vi "Generate Pulse Indexies.vi"(4 "dt":dbl, 5 "Size":i32, 6 "t0":timestamp, 7 "Delay":dbl format="%#_6p", 11 "I-V parameters":T1={"Start magnitude"=0.01, "Magnitude increment"=0.001, "Number of pulses"=8, "Baseline length"=480, "Ramp length"=32, "Top  length"=480, "Threshold "=1e-05, "Processing Delay"=255, "Valhalla range"=0.001, "Interpolation"=64} {"Valhalla range" format="%#_6pA"; "Processing Delay" format="%dpts"; "Threshold" format="%#_6pV"; "Top  length" format="%dpts"; "Ramp length" format="%dpts"; "Baseline length" format="%dpts"; "Magnitude increment" format="%#_6pA"; "Start magnitude" format="%#_6pA"}) -> (3 "Pulse indexies out":T2[](array[typedef]))   [LabVIEW 2016]
uses:
  Pulse indexies.ctl
  I-V parameters.ctl
panel:
  out "32bit integer 2":i32
  out "result":i32
  out "32bit integer":T3
  in  "Pulse indexies":T2
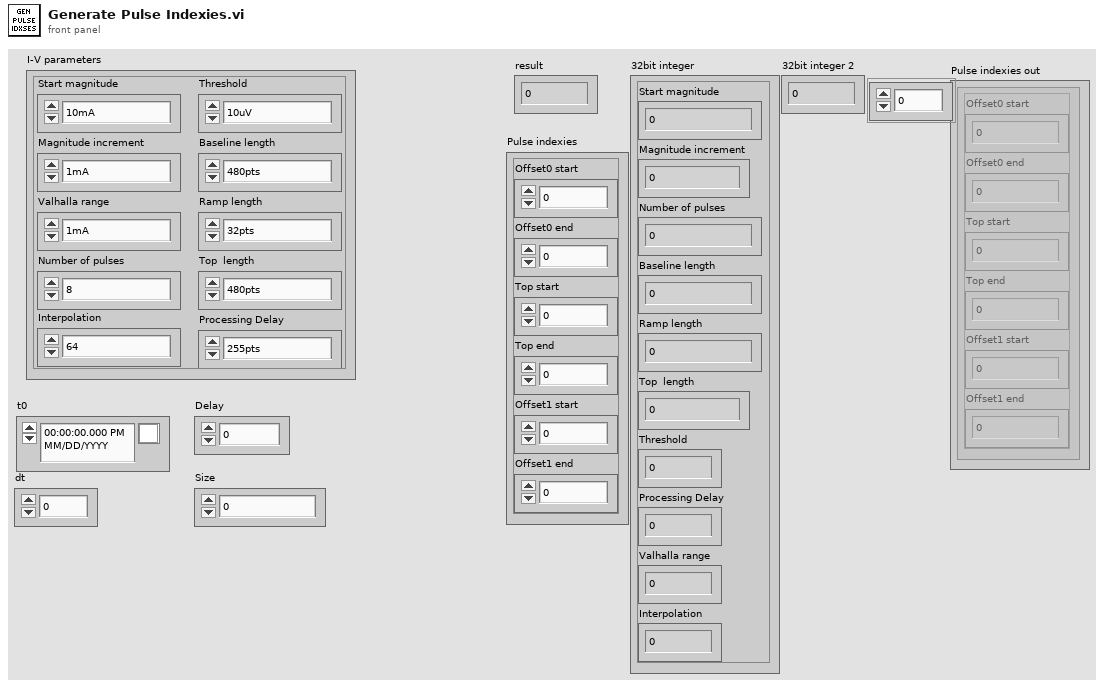
[diagram p1: front panel]
types:
  T1 = typedef "I-V parameters.ctl" = cluster{"Start magnitude":dbl, "Magnitude increment":dbl, "Number of pulses":i32, "Baseline length":i32, "Ramp length":i32, "Top  length":i32, "Threshold ":dbl, "Processing Delay":u16, "Valhalla range":dbl, "Interpolation":i32}
  T2 = typedef "Pulse indexies.ctl" = cluster{"Offset0 start ":i32, "Offset0 end":i32, "Top start":i32, "Top end":i32, "Offset1 start":i32, "Offset1 end":i32}
  T3 = cluster{"Start magnitude":i32, "Magnitude increment":i32, "Number of pulses":i32, "Baseline length":i32, "Ramp length":i32, "Top  length":i32, "Threshold ":i32, "Processing Delay":i32, "Valhalla range":i32, "Interpolation":i32}
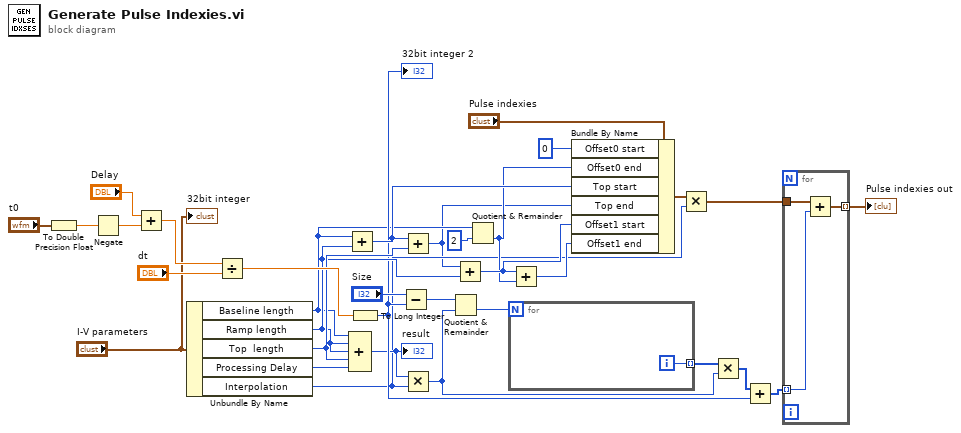
[diagram p0: block diagram]
diagram:
  n1 = To Double Precision Float(number="t0") -> (double precision float=w32:dbl)
  n2 = Negate(x=w32) -> (-x=w31:dbl)
  n3 = Add(x="Delay", y=w31) -> (x+y=w29:dbl)
  n4 = Unbundle By Name("I-V parameters") -> ("Baseline length"=w7:i32, "Ramp length"=w19:i32, "Top  length"=w20:i32, "Processing Delay"=w4:u16, "Interpolation"=w2:i32)
  n5 = Divide(x=w29, y="dt") -> (x/y=w28:dbl)
  n6 = Add(x=w7, y=w19) -> (x+y=w21:i32)
  n7 = Compound Arithmetic op=ADD(w7, w19, w19, w20, w4) -> (w3:i32)
  "result" <- w3
  n8 = To Long Integer(number=w28) -> (32bit integer=w15:i32)
  "32bit integer 2" <- w15
  n9 = Subtract(x="Size", y=w15) -> (x-y=w26:i32)
  n10 = Add(x=w21, y=w20) -> (x+y=w1:i32)
  n11 = Multiply(x=w3, y=w2) -> (x*y=w8:i32)
  n12 = Quotient & Remainder(x=w26, y=w8) -> (floor(x/y)=w25:i32)  [unwired: 1 out]
  n13 = Add(x=w1, y=w19) -> (x+y=w18:i32)
  n14 = Quotient & Remainder(x=w7, y=2) -> (floor(x/y)=w6:i32)  [unwired: 1 out]
  n15 = for {
    N: w25 -> [_]
    tunnel: [w34] -> w16 mode=indexing
    i -> [w34]
  }
  n16 = Add(x=w18, y=w6) -> (x+y=w17:i32)
  n17 = Bundle By Name(cluster="Pulse indexies", "Offset0 start"=0, "Offset0 end"=w6, "Top start"=w21, "Top end"=w1, "Offset1 start"=w18, "Offset1 end"=w17) -> (w9:T2)
  n18 = Multiply(x=w9, y=w2) -> (x*y=w10:T2)
  n19 = Multiply(x=w16, y=w8) -> (x*y=w14:i32[])
  n20 = Add(x=w14, y=w15) -> (x+y=w13:i32[])
  n21 = for {
    tunnel: w13 -> [w37] mode=indexing
    tunnel: w10 -> [w36]
    tunnel: [w35] -> w12 mode=indexing
    n22 = Add(x=w36, y=w37) -> (x+y=w35:T2)
  }
  "Pulse indexies out" <- w12
  "32bit integer" <- "I-V parameters"
